vi "Prueba2.vi"() -> ()   [LabVIEW 2014, in "AD4212C Lib.lvlib"]
uses:
  AD4212C Lib.lvlib
  Typedef/Connection Data.ctl
panel:
  out "x-y":dbl
  out "notification":dbl format="%#_6f"
  in  "VISA resource name Out":T1={"Conection Data"="COM4"}
  in  "stop 2":bool
  in  "stop":bool
  out "error out":errorcluster
  out "VISA resource name Out":T1={"Conection Data"="COM4"}
  in  "error in (no error)":errorcluster
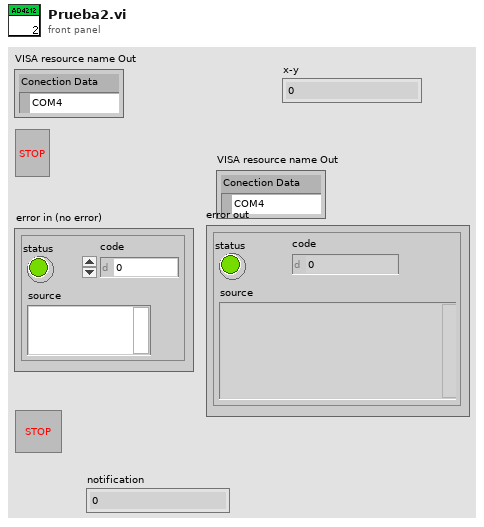
[diagram p1: front panel]
types:
  T1 = typedef "AD4212C Lib.lvlib/Connection Data.ctl" = cluster{"Conection Data":refnum<visa-resource-name>}
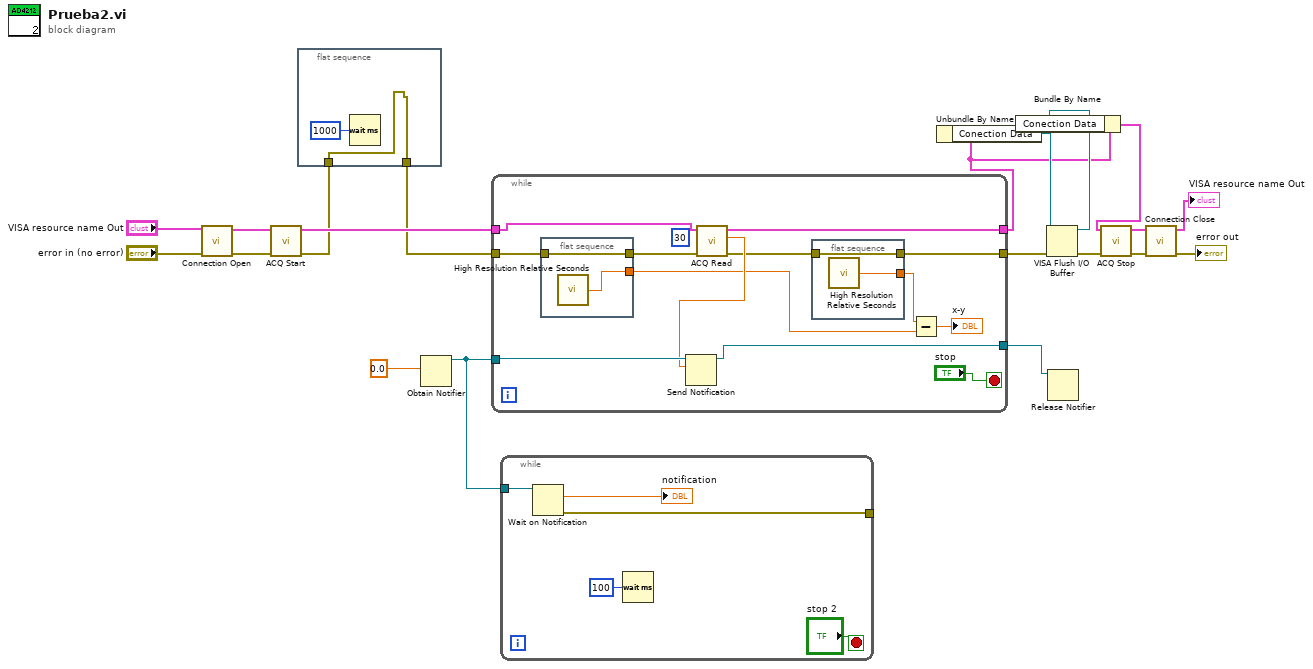
[diagram p0: block diagram]
diagram:
  n1 = call "Connection Open.vi"("VISA resource name Out 3"="VISA resource name Out", "error in (no error)"="error in (no error)") -> ("VISA resource name Out 2"=w20:T1, "error out"=w19:errorcluster)  [unwired: 7 in]
  n2 = call "ACQ Start.vi"("error in (no error)"=w19, "VISA resource name In"=w20) -> ("error out"=w9:errorcluster, "VISA resource name Out"=w13:T1)  [unwired: 8 in]
  n3 = flat-sequence {
    tunnel: w9 -> [w21]
    tunnel: [w21] -> w8
    frame #0 {
      n4 = Wait (ms)(milliseconds to wait=u32 1000) -> ()  [unwired: 1 out]
    }
  }
  n5 = Obtain Notifier(notification data type=0.0) -> (notifier out=w11:refnum<notifier>)  [unwired: 3 in, 2 out]
  n6 = while {
    tunnel: w13 -> [w25]
    tunnel: [w33] -> w3
    tunnel: w8 -> [w31]
    tunnel: [w29] -> w12
    tunnel: w11 -> [w34]
    tunnel: [w23] -> w1
    stop <- "stop" stop-if-true
    (unwired) u32 30 ("byte count")
    n7 = flat-sequence {
      tunnel: w31 -> [w38]
      tunnel: [w39] -> w27
      tunnel: [w38] -> w24
      frame #0 {
        n8 = call <vilib>:"High Resolution Relative Seconds.vi"() -> ("relative seconds"=w39:dbl)
      }
    }
    n9 = call "ACQ Read.vi"("error in (no error)"=w24, "VISA resource name In"=w25) -> ("error out"=w30:errorcluster, "Value"=w32:sgl, "VISA resource name Out"=w33:T1)  [unwired: 7 in]
    n10 = Send Notification(notification=w32, notifier=w34) -> (notifier out=w23:refnum<notifier>)  [unwired: 1 in, 1 out]
    n11 = flat-sequence {
      tunnel: [w37] -> w28
      tunnel: w30 -> [w36]
      tunnel: [w36] -> w29
      frame #0 {
        n12 = call <vilib>:"High Resolution Relative Seconds.vi"() -> ("relative seconds"=w37:dbl)
      }
    }
    n13 = Subtract(x=w28, y=w27) -> (x-y=→"x-y":dbl)
  }
  n14 = while {
    tunnel: w11 -> [w43]
    tunnel: [w40] -> _
    stop <- "stop 2" stop-if-true
    n15 = Wait on Notification(notifier=w43) -> (notification=→"notification":dbl, error out=w40:errorcluster)  [unwired: 3 in, 2 out]
    n16 = Wait (ms)(milliseconds to wait=u32 100) -> ()  [unwired: 1 out]
  }
  n17 = Unbundle By Name(w3) -> ("Conection Data"=w5:refnum<visa-resource-name>)
  n18 = VISA Flush I/O Buffer(VISA resource name=w5, error in (no error)=w12) -> (VISA resource name out=w4:refnum<visa-resource-name>, error out=w14:errorcluster)  [unwired: 1 in]
  n19 = Bundle By Name(cluster=w3, "Conection Data"=w4) -> (w2:T1)
  n20 = Release Notifier(notifier=w1) -> ()  [unwired: 2 in, 3 out]
  n21 = call "ACQ Stop.vi"("error in (no error)"=w14, "VISA resource name In"=w2) -> ("error out"=w17:errorcluster, "VISA resource name Out"=w18:T1)  [unwired: 8 in]
  n22 = call "Connection Close.vi"("error in (no error)"=w17, "VISA resource name In"=w18) -> ("error out"=→"error out":errorcluster, "VISA resource name Out"=→"VISA resource name Out":T1)  [unwired: 8 in]
